vi "XML readSamplesFromXML.getIMValues.vi"(10 "Sample XML":string, 11 "Sample in":T1) -> (3 "Sample out":T1)   [LabVIEW 2011]
uses:
  Controls/PIM.API.Response.Samples.ctl
  iQA Sweep Behavior.ctl
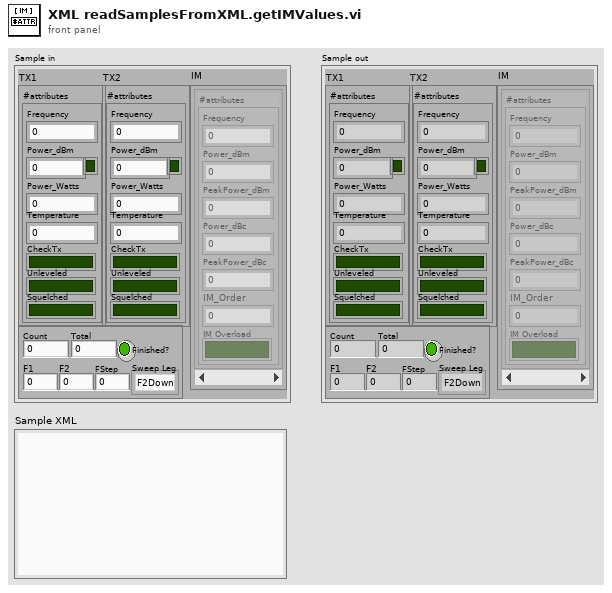
[diagram p1: front panel]
types:
  T1 = typedef "PIM.API.Response.Samples.ctl" = cluster{"TX1":cluster{"#attributes":cluster{"Frequency":dbl, "Power_dBm":dbl, "Power_Watts":dbl, "CheckTx":bool, "Unleveled":bool, "Squelched":bool, "Temperature":dbl, "ToneOn":bool}}, "TX2":cluster{"#attributes":cluster{"Frequency":dbl, "Power_dBm":dbl, "Power_Watts":dbl, "CheckTx":bool, "Unleveled":bool, "Squelched":bool, "Temperature":dbl, "ToneOn":bool}}, "IM":cluster{"#attributes":cluster{"Frequency":dbl, "Power_dBm":dbl, "PeakPower_dBm":dbl, "Power_dBc":dbl, "PeakPower_dBc":dbl, "IM_Order":u8, "IM Overload":bool}}[], "#attributes":cluster{"Count":u32, "Total":u32, "Finished?":bool, "Sweep Leg":T2, "F1":dbl, "F2":dbl, "FStep":dbl}}
  T2 = typedef "iQA Sweep Behavior.ctl" = enum16{"F2Down", "F1Up", "RxMultiIM"}
  T3 = cluster{"#attributes":cluster{"Frequency":dbl, "Power_dBm":dbl, "PeakPower_dBm":dbl, "Power_dBc":dbl, "PeakPower_dBc":dbl, "IM_Order":u8, "IM Overload":bool}}
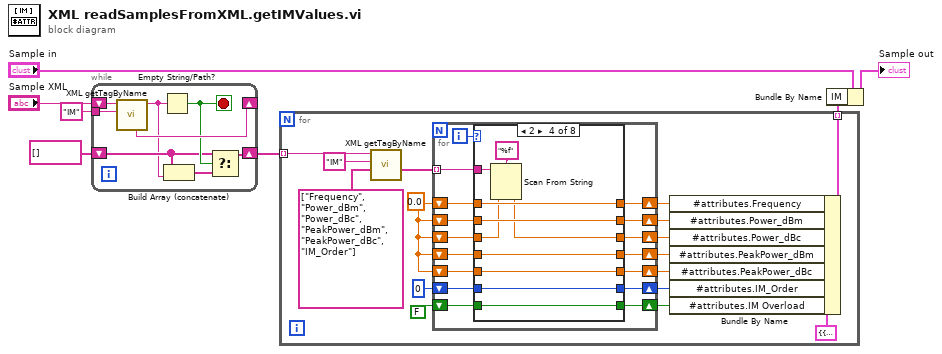
[diagram p0: block diagram]
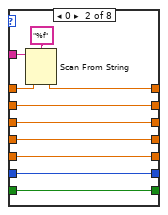
[diagram p3: hidden frame]
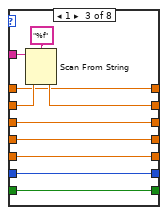
[diagram p4: hidden frame]
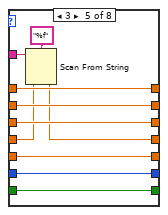
[diagram p5: hidden frame]
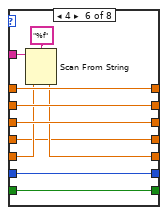
[diagram p6: hidden frame]
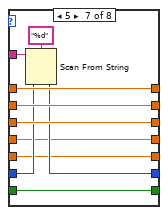
[diagram p7: hidden frame]
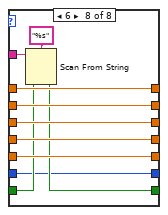
[diagram p8: hidden frame]
diagram:
  n1 = while {
    tunnel: "IM" ("proper case string") -> [w14]
    shift-right: [w12] -> w6
    shift-left: string[] [] -> [w10]
    shift-right: [w13] -> _
    shift-left: "Sample XML" -> [w15]
    stop <- w11 stop-if-true
    n2 = call "XML getTagByName.vi"("Tag Name"=w14, "XML String"=w15) -> ("Matching Tag"=w8:string, "After Tag"=w13:string)  [unwired: 5 in, 3 out]
    n3 = Empty String/Path?(string/path=w8) -> (empty?=w11:bool)
    n4 = Build Array (concatenate)(w10, w8) -> (w9:string[])
    n5 = Select(t=w10, s=w11, f=w9) -> (s? t:f=w12:string[])
  }
  n6 = for {
    tunnel: w6 -> [w22] mode=indexing
    tunnel: [w16] -> w3 mode=indexing
    w20 = 0.0
    n7 = call "XML getTagByName.vi"("Get Attributes"=string[] ["Frequency", "Power_dBm", "Power_dBc", "PeakPower_dBm", "PeakPower_dBc", "IM_Order"], "Tag Name"="IM", "XML String"=w22) -> ("Attribute Values"=w31:string[])  [unwired: 4 in, 4 out]
    n8 = for {
      shift-right: [w46] -> w29
      shift-left: w20 -> [w43]
      shift-right: [w45] -> w28
      shift-left: w20 -> [w44]
      shift-right: [w41] -> w27
      shift-left: w20 -> [w42]
      tunnel: w31 -> [w40] mode=indexing
      shift-right: [w36] -> w26
      shift-left: w20 -> [w39]
      shift-right: [w35] -> w25
      shift-left: w20 -> [w38]
      shift-right: [w34] -> w24
      shift-left: 0 -> [w37]
      shift-right: [w32] -> w18
      shift-left: FALSE -> [w33]
      i -> [w47]
      n9 = case shown="2" w47 {
        tunnel: [w54 w63 w70 w82 w92 w102 w112 w122] -> w46
        tunnel: [w53 w61 w73 w83 w93 w103 w113 w123] -> w45
        tunnel: w44 -> [w53 w61 w72 w83 w93 w103 w113 w123]
        tunnel: w43 -> [w54 w62 w70 w82 w92 w102 w112 w122]
        tunnel: w42 -> [w52 w60 w71 w81 w90 w100 w110 w120]
        tunnel: [w52 w60 w71 w80 w90 w100 w110 w120] -> w41
        tunnel: w40 -> [_ w59 w69 w79 w91 w101 w111 w121]
        tunnel: w39 -> [w51 w58 w68 w78 w89 w97 w107 w119]
        tunnel: w38 -> [w50 w57 w67 w77 w87 w99 w106 w118]
        tunnel: w37 -> [w49 w56 w66 w76 w86 w96 w109 w115]
        tunnel: [w51 w58 w68 w78 w88 w97 w107 w119] -> w36
        tunnel: [w50 w57 w67 w77 w87 w98 w106 w118] -> w35
        tunnel: [w49 w56 w66 w76 w86 w96 w108 w115] -> w34
        tunnel: w33 -> [w48 w55 w65 w75 w85 w95 w105 w117]
        tunnel: [w48 w55 w65 w75 w85 w95 w105 w116] -> w32
        frame Default {
        }
        frame 0 {
          n10 = Scan From String(format string="%f", input string=w59, default 1=w62) -> (output 1=w63:dbl)  [unwired: 2 in, 3 out]
        }
        frame 1 {
          n11 = Scan From String(format string="%f", input string=w69, default 1=w72) -> (output 1=w73:dbl)  [unwired: 2 in, 3 out]
        }
        frame 2 {
          n12 = Scan From String(format string="%f", input string=w79, default 1=w81) -> (output 1=w80:dbl)  [unwired: 2 in, 3 out]
        }
        frame 3 {
          n13 = Scan From String(format string="%f", input string=w91, default 1=w89) -> (output 1=w88:dbl)  [unwired: 2 in, 3 out]
        }
        frame 4 {
          n14 = Scan From String(format string="%f", input string=w101, default 1=w99) -> (output 1=w98:dbl)  [unwired: 2 in, 3 out]
        }
        frame 5 {
          n15 = Scan From String(format string="%d", input string=w111, default 1=w109) -> (output 1=w108:i32)  [unwired: 2 in, 3 out]
        }
        frame 6 {
          n16 = Scan From String(format string="%s", input string=w121, default 1=w117) -> (output 1=w116:bool)  [unwired: 2 in, 3 out]
        }
      }
    }
    n17 = Bundle By Name(cluster=T3 {"#attributes"={"Frequency"=0.0, "Power_dBm"=0.0, "PeakPower_dBm"=0.0, "Power_dBc"=0.0, "PeakPower_dBc"=0.0, "IM_Order"=0, "IM Overload"=FALSE}} ("IM"), "#attributes.Frequency"=w29, "#attributes.Power_dBm"=w28, "#attributes.Power_dBc"=w27, "#attributes.PeakPower_dBm"=w26, "#attributes.PeakPower_dBc"=w25, "#attributes.IM_Order"=w24, "#attributes.IM Overload"=w18) -> (w16:T3)
  }
  n18 = Bundle By Name(cluster="Sample in", "IM"=w3) -> (→"Sample out":T1)
